vi "ObtainBroadcastEvents.vi"(7 "Init? (f)":bool, 8 "error in (no error)":errorcluster) -> (0 "error out":errorcluster, 2 "clBroadcastEvents":T1)   [LabVIEW 2014, in "WfrmModule.lvlib"]
uses:
  WfrmModule.lvlib
  clBroadcastEvents.ctl
  clEventType.ctl
panel:
  # "These are the default\nBroadcast Events\nfor the cloneable module\n\nIf you want to add your own,create the typedefs in the PublicAPI/Arguments/Broadcast foldr and add event references to the clBroadcastEvents typedef in the Private/Broadcast folder."
  # "If you want to add other Broadcast Events, open this typedef, copy an existing event and rename it to your event name.\n\nNext create a typedef for the  data and put it into PublicAPI/Arguments/Broadcasts"
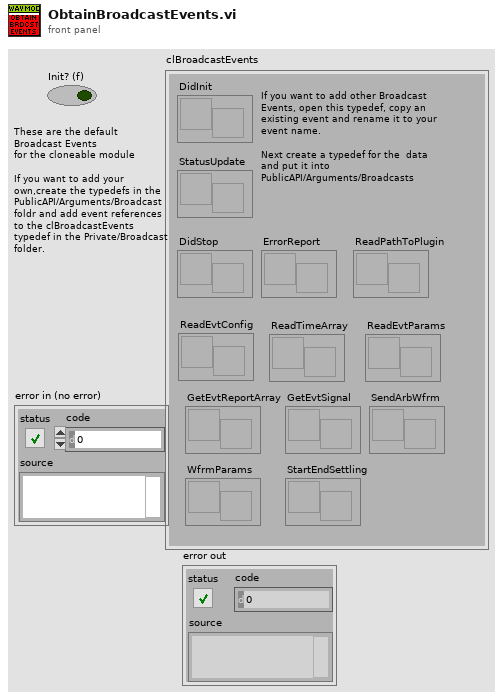
[diagram p1: front panel]
types:
  T1 = typedef "WfrmModule.lvlib/clBroadcastEvents.ctl" = cluster{"DidInit":refnum<user-event>, "StatusUpdate":refnum<user-event>, "ErrorReport":refnum<user-event>, "DidStop":refnum<user-event>, "ReadEvtConfig":refnum<user-event>, "ReadTimeArray":refnum<user-event>, "ReadEvtParams":refnum<user-event>, "GetEvtReportArray":refnum<user-event>, "ReadPathToPlugin":refnum<user-event>, "GetEvtSignal":refnum<user-event>, "SendArbWfrm":refnum<user-event>, "WfrmParams":refnum<user-event>, "StartEndSettling":refnum<user-event>}
  T2 = typedef "WfrmModule.lvlib/clEventType.ctl" = cluster{"ModuleID":i32, "Data":variant}
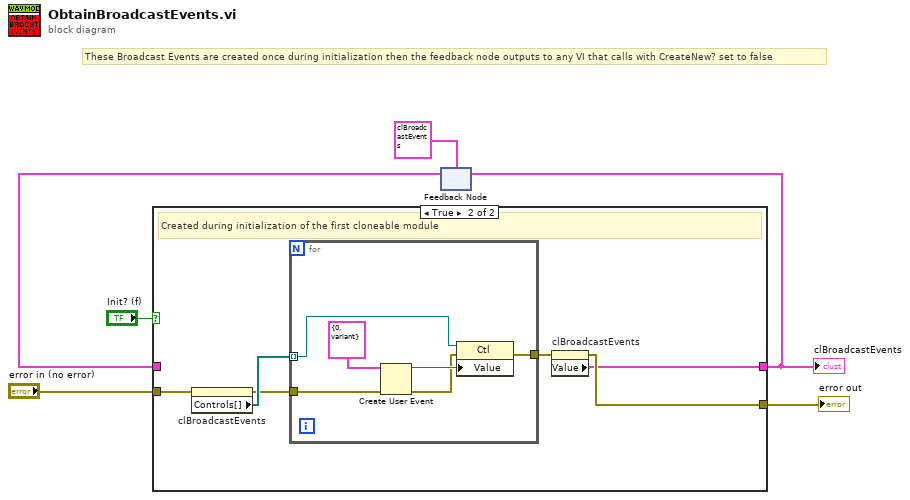
[diagram p0: block diagram]
diagram:
  # "These Broadcast Events are created once during initialization then the feedback node outputs to any VI that calls with CreateNew? set to false"
  n1 = feedback #1(T1 {"DidInit"=refnum, "StatusUpdate"=refnum, "ErrorReport"=refnum, "DidStop"=refnum, "ReadEvtConfig"=refnum, "ReadTimeArray"=refnum, "ReadEvtParams"=refnum, "GetEvtReportArray"=refnum, "ReadPathToPlugin"=refnum, "GetEvtSignal"=refnum, "SendArbWfrm"=refnum, "WfrmParams"=refnum, "StartEndSettling"=refnum} ("Value")) -> (w2:T1)
  n2 = case shown="True" "Init? (f)" {
    tunnel: "error in (no error)" -> [w7 w10]
    tunnel: [w7 w14] -> w5
    tunnel: [w8 w13] -> w4
    tunnel: w2 -> [w8 _]
    frame False {
      # "Modules can register to receive these broadcasts or subesquenc cloneable modules can get the events here"
    }
    frame True {
      # "Created during initialization of the first cloneable module"
      n3 = property on="clBroadcastEvents" class="Clust (strict)"(error in=w10) -> (error out=w9:errorcluster, "Controls[]"=w11:refnum<vi>[])  [unwired: 1 in, 1 out]
      n4 = for {
        tunnel: w11 -> [w15] mode=indexing
        tunnel: w9 -> [w20]
        tunnel: [w18] -> w12
        n5 = Create User Event(user event datatype=T2 {"ModuleID"=0, "Data"=variant} ("clBroadcast"), error in=w20) -> (user event=w19:refnum<user-event>, error out=w17:errorcluster)
        n6 = property class="Ctl"(reference=w15, error in=w17, "Value"=w19) -> (error out=w18:errorcluster)  [unwired: 1 out]
      }
      n7 = property on="clBroadcastEvents" class="Clust (strict)"(error in=w12) -> (error out=w14:errorcluster, "Value"=w13:T1)  [unwired: 1 in, 1 out]
    }
  }
  "error out" <- w5
  "clBroadcastEvents" <- w4
  n8 = feedback-in #1(w4) -> ()
